vi "test control.vi"(0 "Test Controls":T1 {"Lift" scale=-1.0..1.0; "Arm" scale=-1.0..1.0; "Drive Train Z" scale=-1.0..1.0; "Drive Train Y" scale=-1.0..1.0; "Drive Train X" scale=-1.0..1.0}) -> ()   [LabVIEW 2015]
uses:
  <vilib>/Rock Robotics/Network Tables/NT Write Boolean Array.vi
  <vilib>/Rock Robotics/Network Tables/NT Write Numeric Array.vi
panel:
  # "Drive Encoders"
  # "Other Encoders"
  # "Manual Override"
  # "Joystick Control"
  # "For Joystick Control\nManual Override Option: Use the above controls \n (Manual Override).\nManual: Use the joystick for manual control.\nDisable: Disable the motor output.\n\nFor Encoder Control\nThe encoder buttons reset/home the encoders."
  # "Gyroscope"
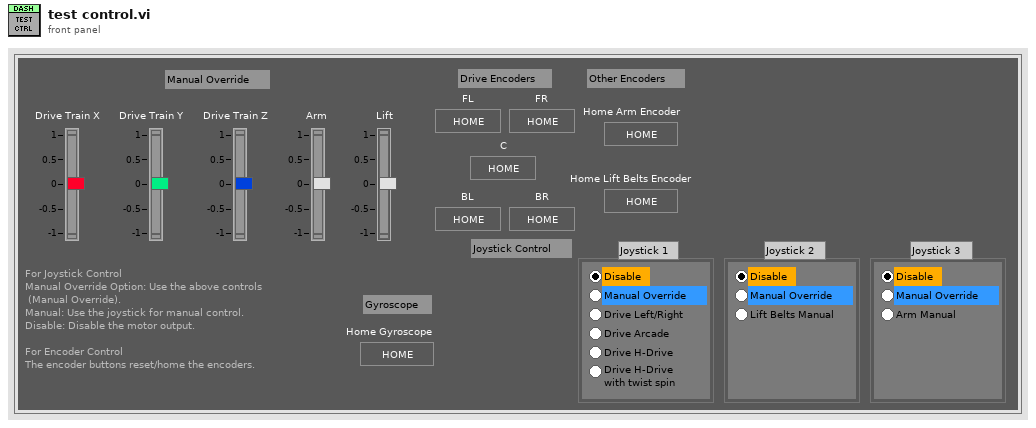
[diagram p1: front panel]
types:
  T1 = cluster{"Drive Train X":dbl, "Drive Train Y":dbl, "Drive Train Z":dbl, "Arm":dbl, "Lift":dbl, "FL":bool, "FR":bool, "BL":bool, "BR":bool, "C":bool, "Home Arm Encoder":bool, "Home Lift Belts Encoder":bool, "Joystick 1":enum32{"Disable", "Drive Left/Right", "Drive Arcade", "Drive H-Drive", "Drive H-Drive \nwith twist spin", "Manual Override"}, "Joystick 2":enum32{"Disable", "Lift Belts Manual", "Manual Override"}, "Joystick 3":enum32{"Disable", "Arm Manual", "Manual Override"}, "Home Gyroscope":bool}
  T2 = enum32{"Disable", "Drive Left/Right", "Drive Arcade", "Drive H-Drive", "Drive H-Drive \nwith twist spin", "Manual Override"}
  T3 = enum32{"Disable", "Lift Belts Manual", "Manual Override"}
  T4 = enum32{"Disable", "Arm Manual", "Manual Override"}
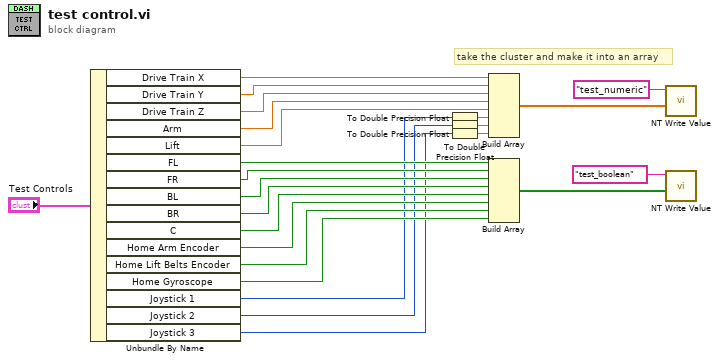
[diagram p0: block diagram]
diagram:
  # "take the cluster and make it into an array"
  n1 = Unbundle By Name("Test Controls") -> ("Drive Train X"=w8:dbl, "Drive Train Y"=w7:dbl, "Drive Train Z"=w6:dbl, "Arm"=w5:dbl, "Lift"=w4:dbl, "FL"=w17:bool, "FR"=w16:bool, "BL"=w15:bool, "BR"=w14:bool, "C"=w13:bool, "Home Arm Encoder"=w12:bool, "Home Lift Belts Encoder"=w11:bool, "Home Gyroscope"=w10:bool, "Joystick 1"=w3:T2, "Joystick 2"=w2:T3, "Joystick 3"=w1:T4)
  n2 = To Double Precision Float(number=w3) -> (double precision float=w22:dbl)
  n3 = To Double Precision Float(number=w2) -> (double precision float=w23:dbl)
  n4 = To Double Precision Float(number=w1) -> (double precision float=w24:dbl)
  n5 = Build Array(w8, w7, w6, w5, w4, w22, w23, w24) -> (w21:dbl[])
  n6 = Build Array(w17, w16, w15, w14, w13, w12, w11, w10) -> (w9:bool[])
  n7 = call-poly <vilib>:"NT Write Value.vi"("Numeric Array"=w21, "Name"="test_numeric") -> ()  [unwired: 9 in, 1 out]
  n8 = call-poly <vilib>:"NT Write Value.vi"("Boolean Array"=w9, "Name"="test_boolean") -> ()  [unwired: 9 in, 1 out]
